vi "validate.vi"(8 "error in":errorcluster, 11 "Special Test configuration":refnum<class "Special Test configuration.lvclass">) -> (0 "error out":errorcluster, 3 "Special Test configuration out":refnum<class "Special Test configuration.lvclass">)   [LabVIEW 2025, in "Special Test.lvlib" / "Special Test configuration.lvclass"]
doc: "Provides an interface for performing validation on a given configuration. Any children should define the behavior of this function to ensure that the configuration in memory can be used by the runtime class.Copyright 2017 National Instruments Corporation\n\nLicensed under the Apache License, Version 2.0 (the \"License\"); you may not use this file except in compliance with the License. You may obtain a copy of the License at http://www.apache.org/licenses/LICENSE-2.0\nUnless required by applicable law or agreed to in writing, software distributed under the License is distributed on an \"AS IS\" BASIS, WITHOUT WARRANTIES OR CONDITIONS OF ANY KIND, either express or implied. See the License for the specific language governing permissions and limitations under the License."
uses:
  Special Test configuration.lvclass
  Special Test configuration.lvclass/Special Test configuration.ctl
  Read Test Info.vi
  Users/Public/Documents/Sandia National Labs/TSS Plugin/CEF.lvlibp
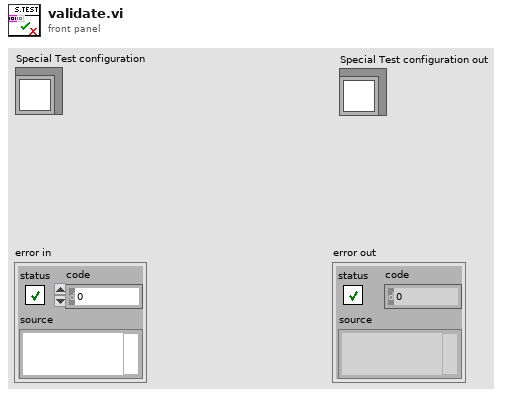
[diagram p1: front panel]
types:
  T1 = typedef "Special Test.lvlib/Special Test configuration.lvclass/Test Info.ctl" = cluster{"General":cluster{"Location":string, "Operator":string}, "Doc":cluster{"Shorthand Test Name":string, "MRS Code":string, "P6 Test Activity Name":string, "Test Plan":string, "Wiring Diagram":string}, "Test Setup":cluster{"Series":string, "Test Code":string, "Test Group":string, "Config Type":string}, "Run":cluster{"Temperature":string, "Voltage":string, "Attempt":u32, "Test Run":string, "Pre-Test Notes":string, "Source Code":string, "During Environment":string, "Enable Dropouts":bool}}
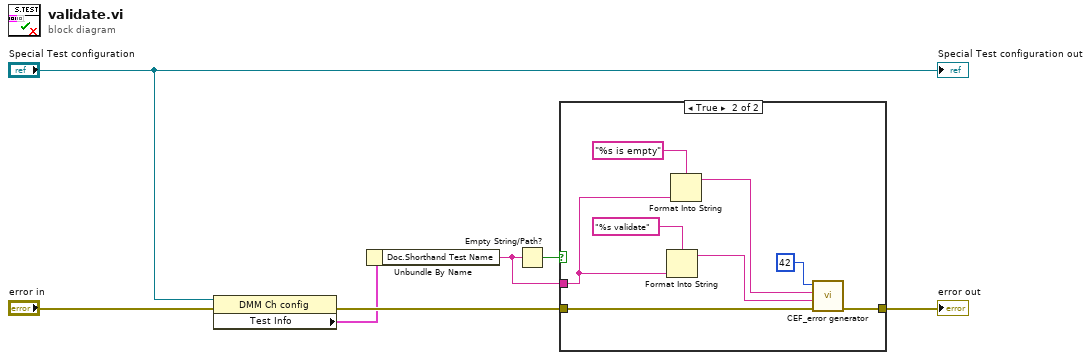
[diagram p0: block diagram]
diagram:
  n1 = property class="DMM Ch config"(reference="Special Test configuration", error in="error in") -> (error out=w5:errorcluster, "Test Info"=w3:T1)  [unwired: 1 out]
  n2 = Unbundle By Name(w3) -> ("Doc.Shorthand Test Name"=w1:string)
  n3 = Empty String/Path?(string/path=w1) -> (empty?=w2:bool)
  n4 = case shown="True" w2 {
    tunnel: w5 -> [w8 w16]
    tunnel: [w8 w15] -> w6
    tunnel: w1 -> [_ w10]
    frame False {
    }
    frame True {
      n5 = Format Into String(format string="%s validate" ("append error message"), w10) -> (resulting string=w9:string)  [unwired: 2 in, 1 out]
      n6 = Format Into String(format string="%s is empty" ("append error message"), w10) -> (resulting string=w12:string)  [unwired: 2 in, 1 out]
      n7 = call "CEF_error generator.vi"("error in"=w16, "source"=w9, "append error message"=w12, "error code (0)"=42) -> ("error out"=w15:errorcluster)  [unwired: 5 in]
    }
  }
  "error out" <- w6
  "Special Test configuration out" <- "Special Test configuration"
